vi "Create Last Temperature Entry.vi"(10 "Channel":string, 11 "Thermometer DAQmx RTD Cont CFG in":refnum<class "Thermometer DAQmx RTD Cont CFG.lvclass">) -> (3 "Thermometer DAQmx RTD Cont CFG out":refnum<class "Thermometer DAQmx RTD Cont CFG.lvclass">)   [LabVIEW 2024, in "Thermometer DAQmx RTD Cont CFG.lvclass"]
uses:
  Thermometer DAQmx RTD Cont CFG.lvclass
  Thermometer DAQmx RTD Cont CFG.lvclass/Thermometer DAQmx RTD Cont CFG.ctl
  <vilib>/Utility/miscctls.llb/LVMapReplaceAction.ctl
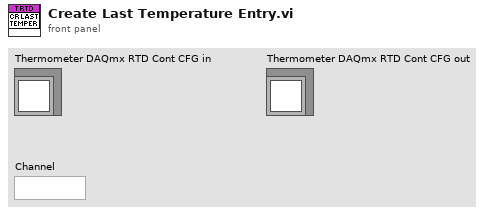
[diagram p1: front panel]
types:
  T1 = typedef "LVMapReplaceAction.ctl" = enum32{"Modify Entry only if found", "Add or Modify Entry", "Delete Entry"}
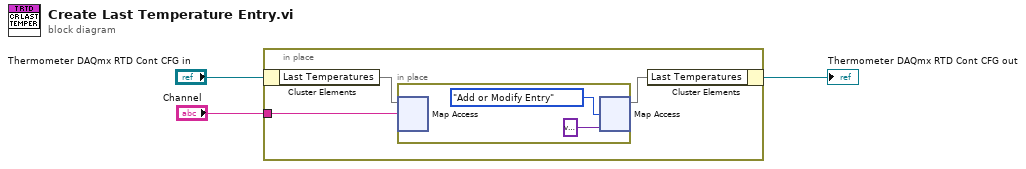
[diagram p0: block diagram]
diagram:
  n1 = in-place {
    in-place-border: "Channel" -> [w6]
    n2 = in-place-cluster #1("Thermometer DAQmx RTD Cont CFG in") -> ("Last Temperatures"=w5:map{string, variant})
    n3 = in-place {
      n4 = in-place-map #2(w5, w6) -> ()  [unwired: 1 in, 2 out]
      n5 = in-place-map #2(variant, LVMapReplaceAction."Add or Modify Entry" ("action")) -> (w4:map{string, variant})  [unwired: 2 out]
    }
    n6 = in-place-cluster #1("Last Temperatures"=w4) -> (→"Thermometer DAQmx RTD Cont CFG out":refnum<class "Thermometer DAQmx RTD Cont CFG.lvclass">)
  }
